vi "PosStrikerAnguloGol.vi"(8 "AnguloAttacker":dbl, 9 "atacando contra":bool, 10 "IA State":T1={"our_robots"=[], "enemy_robots"=[], "balls"=[], "geometry"={"line_width"=0, "field_length"=0, "field_width"=0, "boundary_width"=0, "referee_width"=0, "goal_width"=0, "goal_depth"=0, "goal_wall_width"=0, "center_circle_radius"=0, "defense_radius"=0, "defense_stretch"=0, "free_kick_from_defense_dist"=0, "penalty_spot_from_field_line_dist"=0, "penalty_line_from_spot_dist"=0}, "IA Judge"={"stage"="", "command"="", "our_goalie_id"=0.0, "enemy_goalie_id"=0.0, "command enum"=enum."Halt", "Time"=enum."Azul"}, "Received Timestamp"=timestamp(0 s since 1904-01-01), "Events"={"Touch"=FALSE, "Ball out"=FALSE, "id touch"=0.0, "Ball out of \nVision"=FALSE, "Ball inside \nGoalie area"=FALSE, "Robot not responding"=FALSE, "Robots responding status"=[1.0, 1.0, 1.0, 1.0, 1.0, 1.0], "Enemy Ball \nPossession"=FALSE, "Pass State"=FALSE, "id end of pass"=0.0, "Kick"=FALSE, "Id ini Possession"=0.0, "Ball Possesion"=FALSE, "Id Possesion"=0.0, "Direct Kick"=FALSE}}) -> (2 "theta final":dbl)   [LabVIEW 2017]
uses:
  Core/AI Input.ctl
  Core/AI Robot.ctl
  Intel/Functions Enum.ctl
  Intel/AttackerStates.ctl
  Path Planning/RRT/PathDests.ctl
  Path Planning/RRT/PathDest.ctl
  Core/AI Ball.ctl
  Core/Field Size.ctl
  Core/AI Judge.ctl
  Intel/Command Enum.ctl
  Events/Events.ctl
panel:
  in  "XdoAttacker":dbl
  in  "YdoAttacker":dbl
  in  "Array":dbl[](array[numeric])=[0.0, 0.0, 0.0, 0.0, 0.0, 0.0]
  in  "Contador 2":dbl
  in  "theta2":dbl=-1.57
  in  "inicio do intervalo":dbl=-1.57
  in  "tamanho do intervalo":dbl
  in  "valor de theta":dbl
  in  "RobôsParaAnalisar":dbl[][](array[numeric])=[[99999.0, 99999.0], [99999.0, 99999.0], [99999.0, 99999.0], [99999.0, 99999.0], [99999.0, 99999.0], [99999.0, 99999.0], [99999.0, 99999.0]]
  in  "Contador":dbl
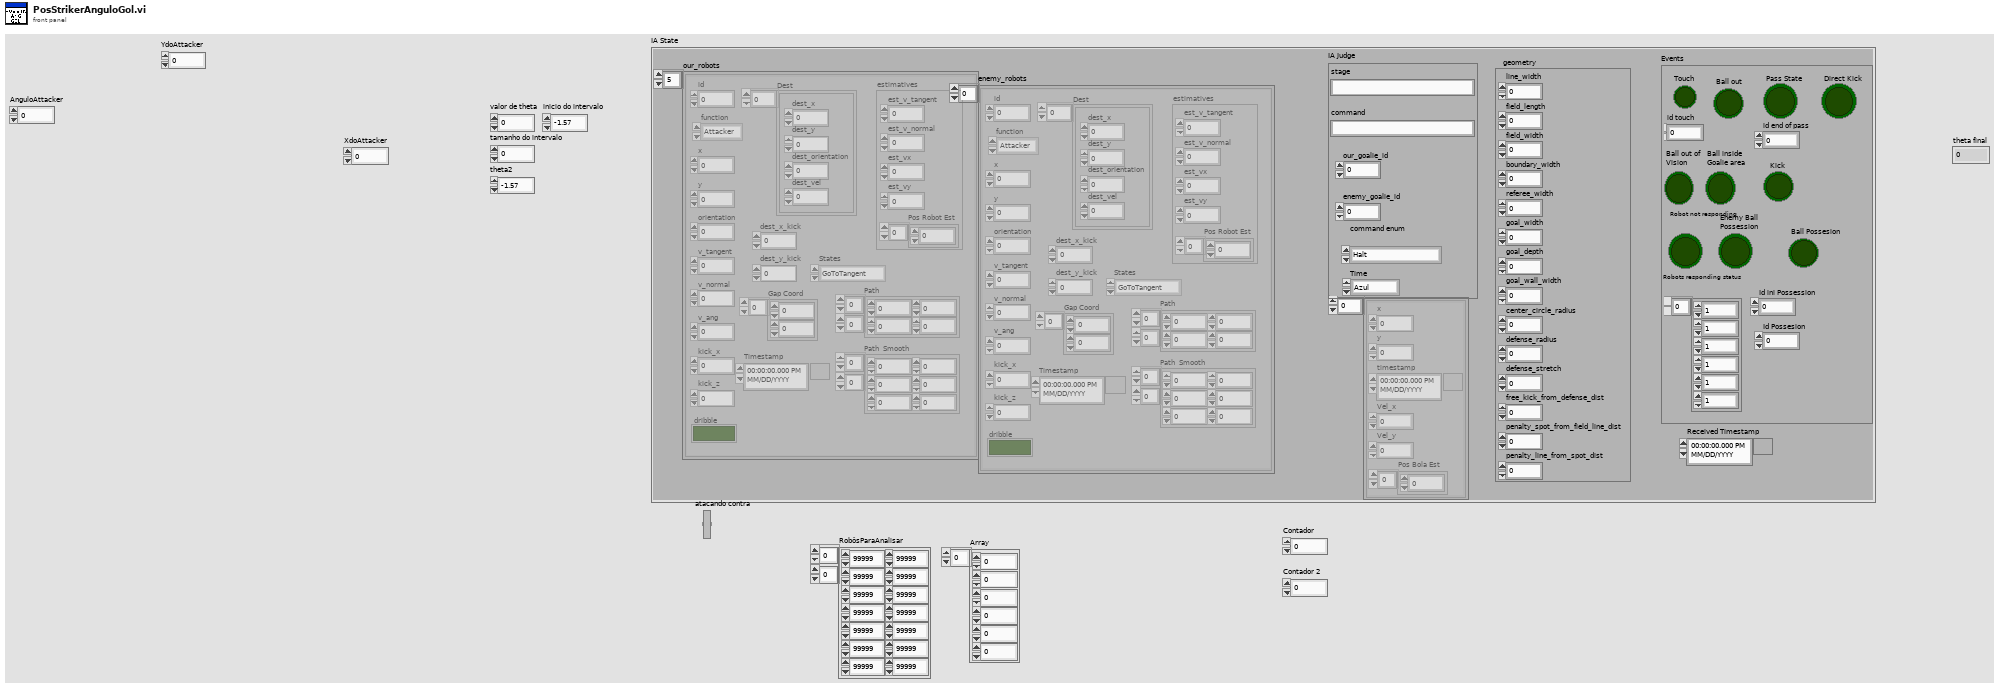
[diagram p1: front panel]
types:
  T1 = typedef "AI Input.ctl" = cluster{"our_robots":T2[], "enemy_robots":T2[], "balls":T7[], "geometry":T8, "IA Judge":T9, "Received Timestamp":timestamp, "Events":T11}
  T2 = typedef "AI Robot.ctl" = cluster{"id":u32, "function":T3, "x":dbl, "y":dbl, "orientation":dbl, "v_tangent":dbl, "v_normal":dbl, "v_ang":dbl, "kick_x":dbl, "kick_z":dbl, "dribble":bool, "Timestamp":timestamp, "estimatives":cluster{"est_v_tangent":dbl, "est_v_normal":dbl, "est_vx":dbl, "est_vy":dbl, "Pos Robot Est":dbl[]}, "dest_x_kick":dbl, "dest_y_kick":dbl, "Gap Coord":dbl[], "States":T4, "Path ":dbl[][], "Path  Smooth":dbl[][], "Dest":T5}
  T3 = typedef "Functions Enum.ctl" = enum16{"Attacker", "Goalie", "Defender", "Striker", "Goto 0", "Dummy", "Kicker", "ZigZag 0", "ZigZag 1", "ZigZag 2", "ZigZag 3", "ZigZag 4", "ZigZag 5", "ZigZag 6", "ZigZag 7", "ZigZag 8", ""}
  T4 = typedef "AttackerStates.ctl" = enum16{"Pass", "GoToTangent", "BallGetting", "GoToKick", ""}
  T5 = typedef "PathDests.ctl" = T6[]
  T6 = typedef "PathDest.ctl" = cluster{"dest_x":dbl, "dest_y":dbl, "dest_orientation":dbl, "dest_vel":dbl}
  T7 = typedef "AI Ball.ctl" = cluster{"x":dbl, "y":dbl, "timestamp":timestamp, "Vel_x":dbl, "Vel_y":dbl, "Pos Bola Est":dbl[]}
  T8 = typedef "Field Size.ctl" = cluster{"line_width":u32, "field_length":u32, "field_width":u32, "boundary_width":u32, "referee_width":u32, "goal_width":u32, "goal_depth":u32, "goal_wall_width":u32, "center_circle_radius":u32, "defense_radius":u32, "defense_stretch":u32, "free_kick_from_defense_dist":u32, "penalty_spot_from_field_line_dist":u32, "penalty_line_from_spot_dist":u32}
  T9 = typedef "AI Judge.ctl" = cluster{"stage":string, "command":string, "our_goalie_id":dbl, "enemy_goalie_id":dbl, "command enum":T10, "Time":enum16{"Azul", "Amarelo"}}
  T10 = typedef "Command Enum.ctl" = enum16{"Halt", "Stop", "Force Start", "PKA Normal Start", "Prepare Kickoff Ally", "PKE Normal Start", "Prepare Kickoff Enemy", "Prepare Penalty Ally", "PPA Normal Start", "Prepare Penalty Enemy", "PPE Normal Start", "Direct Free Enemy", "Direct Free Ally", "Indirect Free Enemy", "Indirect Free Ally", "Timeout Enemy", "Timeout Ally", "Goal Enemy", "Goal Ally", "Ball Placement Enemy", "Ball Placement Ally", "Normal Half Time", "Extra Time Break", "Extra Half Time", "None", "Post Game"}
  T11 = typedef "Events.ctl" = cluster{"Touch":bool, "Ball out":bool, "id touch":dbl, "Ball out of \nVision":bool, "Ball inside \nGoalie area":bool, "Robot not responding":bool, "Robots responding status":dbl[], "Enemy Ball \nPossession":bool, "Pass State":bool, "id end of pass":dbl, "Kick":bool, "Id ini Possession":dbl, "Ball Possesion":bool, "Id Possesion":dbl, "Direct Kick":bool}
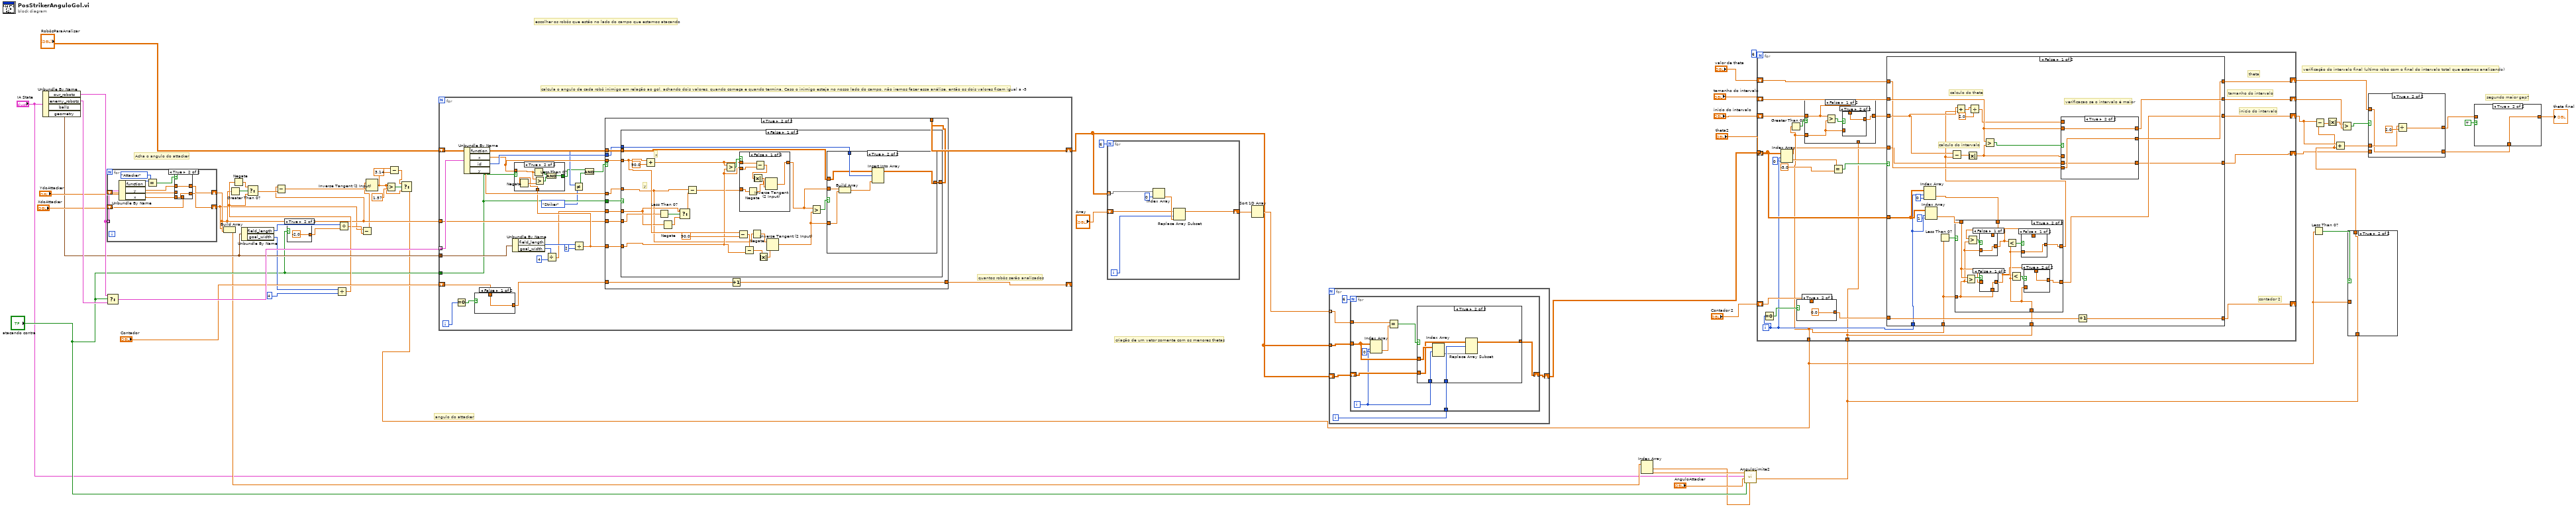
[diagram p0: block diagram]
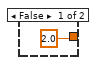
[diagram p4: hidden frame]
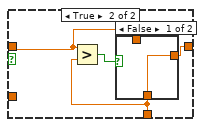
[diagram p9: hidden frame]
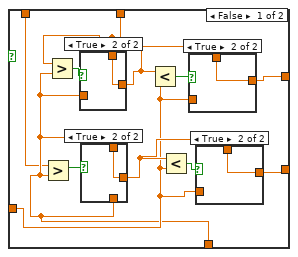
[diagram p12: hidden frame]
diagram:
  # "segundo maior gap?"
  # "verificação do intervalo final (ultimo robo com o final do intervalo total que estamos analisando)"
  # "calcula o angulo de cada robô inimigo em relação ao gol, achando dois valores, quando começa e quando termina. Caso o inimigo esteja no nosso lado do campo, não iremos fazer essa análise, então os dois valores ficam igual a -5"
  # "angulo do attacker"
  # "Acha o angulo do attacker"
  # "criação de um vetor somente com os menores thetas"
  # "escolher os robôs que estão no lado do campo que estamos atacando"
  n1 = Unbundle By Name("IA State") -> ("our_robots"=w37:T2[], "enemy_robots"=w60:T2[], "geometry"=w34:T8)  [unwired: 1 out]
  n2 = for {
    tunnel: w37 -> [w70] mode=indexing
    shift-right: [w65] -> w15
    shift-left: "YdoAttacker" -> [w64]
    shift-right: [w62] -> w14
    shift-left: "XdoAttacker" -> [w61]
    n3 = Unbundle By Name(w70) -> ("function"=w69:T3, "y"=w66:dbl, "x"=w63:dbl)
    n4 = Equal?(x=w69, y=Functions_Enum."Attacker") -> (x = y?=w67:bool)
    n5 = case shown="True" w67 {
      tunnel: w66 -> [_ w74]
      tunnel: [w72 w74] -> w65
      tunnel: w64 -> [w72 _]
      tunnel: w63 -> [_ w73]
      tunnel: [w71 w73] -> w62
      tunnel: w61 -> [w71 _]
      frame False {
      }
      frame True {
      }
    }
  }
  n6 = Select(t=w37, s="atacando contra", f=w60) -> (s? t:f=w59:T2[])
  n7 = Build Array(w14, w15) -> (w13:dbl[])
  n8 = Greater Than 0?(x=w15) -> (x > 0?=w30:bool)
  n9 = Unbundle By Name(w34) -> ("field_length"=w31:u32, "goal_width"=w33:u32)
  n10 = case shown="True" "atacando contra" {
    tunnel: [2.0 ("y") -2.0 ("y")] -> w25
    frame False {
    }
    frame True {
    }
  }
  n11 = Divide(x=w33, y=u32 4) -> (x/y=w28:dbl)
  n12 = Negate(x=w28) -> (-x=w29:dbl)
  n13 = Select(t=w29, s=w30, f=w28) -> (s? t:f=w27:dbl)
  n14 = Subtract(x=w15, y=w27) -> (x-y=w2:dbl)
  n15 = Divide(x=w31, y=w25) -> (x/y=w26:dbl)
  n16 = Subtract(x=w14, y=w26) -> (x-y=w1:dbl)
  n17 = Inverse Tangent (2 Input)(1:w2, 2:w1) -> (0:w4:dbl)
  n18 = Greater?(x=w4, y=1.57) -> (0:w7:bool)
  n19 = Subtract(x=w4, y=3.14) -> (x-y=w5:dbl)
  n20 = Select(t=w5, s=w7, f=w4) -> (s? t:f=w3:dbl)
  n21 = for {
    tunnel: w59 -> [w101] mode=indexing
    tunnel: "atacando contra" -> [w83]
    shift-right: [w91] -> w47
    shift-left: "RobôsParaAnalisar" -> [w100]
    shift-right: [w92] -> _
    shift-left: "Contador" -> [w94]
    tunnel: w34 -> [w84]
    tunnel: w15 -> [w88]
    i -> [w95]
    # "quantos robôs serão analisados"
    n22 = Equal To 0?(x=w95) -> (x = 0?=w96:bool)
    n23 = Unbundle By Name(w101) -> ("function"=w81:T3, "x"=w98:dbl, "id"=w99:u32, "y"=w97:dbl)
    n24 = case shown="False" w96 {
      tunnel: w94 -> [w102 _]
      tunnel: [w102 0.0] -> w93
      frame False {
      }
      frame True {
      }
    }
    n25 = Unbundle By Name(w84) -> ("field_length"=w90:u32, "goal_width"=w87:u32)
    n26 = Divide(x=w87, y=u32 4) -> (x/y=w85:dbl)
    n27 = Not Equal?(x=w81, y=Functions_Enum."Striker") -> (x != y?=w78:bool)
    n28 = Divide(x=w90, y=u32 2) -> (x/y=w89:dbl)
    n29 = case shown="True" w83 {
      tunnel: w98 -> [w108 w109]
      tunnel: [w104 w114] -> w77
      tunnel: w89 -> [w107 w110]
      frame False {
        n30 = Less?(x=w108, y=w107) -> (x < y?=w105:bool)
        n31 = Greater Than 0?(x=w108) -> (x > 0?=w106:bool)
        n32 = And(x=w106, y=w105) -> (x .and. y?=w104:bool)
      }
      frame True {
        n33 = Negate(x=w110) -> (-x=w111:dbl)
        n34 = Less Than 0?(x=w109) -> (x < 0?=w113:bool)
        n35 = Greater?(x=w109, y=w111) -> (0:w112:bool)
        n36 = And(x=w113, y=w112) -> (x .and. y?=w114:bool)
      }
    }
    n37 = And(x=w77, y=w78) -> (x .and. y?=w79:bool)
    n38 = case shown="True" w79 {
      tunnel: w100 -> [w119 w126]
      tunnel: w99 -> [w118 w124]
      tunnel: w98 -> [_ w128]
      tunnel: w97 -> [_ w125]
      tunnel: w93 -> [w120 w130]
      tunnel: [w120 w131] -> w92
      tunnel: [w115 w123] -> w91
      tunnel: w83 -> [_ w129]
      tunnel: w89 -> [_ w127]
      tunnel: w88 -> [_ w122]
      tunnel: w85 -> [_ w121]
      frame False {
        w117 = -5.0 ("element")
        n39 = Build Array(w117, w117) -> (w116:dbl[])
        n40 = Insert Into Array(array=w119, index (row)=w118, new element=w116) -> (w115:dbl[][])  [unwired: 1 in]
      }
      frame True {
        n41 = case shown="False" w129 {
          tunnel: w128 -> [w144 w193]
          tunnel: w127 -> [w143 w196]
          tunnel: w126 -> [w145 w188]
          tunnel: w125 -> [w133 w177]
          tunnel: w124 -> [w146 w187]
          tunnel: [w142 w184] -> w123
          tunnel: w122 -> [w137 w181]
          tunnel: w121 -> [w136 w178]
          frame False {
            # "y"
            # "x"
            n42 = Add(x=w144, y=90.0) -> (x+y=w152:dbl)
            n43 = Less Than 0?(x=w137) -> (x < 0?=w140:bool)
            n44 = Negate(x=w136) -> (-x=w139:dbl)
            n45 = Select(t=w136, s=w140, f=w139) -> (s? t:f=w138:dbl)
            n46 = Subtract(x=w133, y=w138) -> (x-y=w135:dbl)
            n47 = Greater?(x=w152, y=w143) -> (0:w153:bool)
            n48 = Subtract(x=w144, y=90.0) -> (x-y=w150:dbl)
            n49 = case shown="False" w153 {
              tunnel: w152 -> [w173 _]
              tunnel: [w171 1.57] -> w148
              tunnel: w143 -> [w172 _]
              tunnel: w135 -> [w167 _]
              frame False {
                n50 = Negate(x=w167) -> (-x=w168:dbl)
                n51 = Subtract(x=w173, y=w172) -> (x-y=w170:dbl)
                n52 = Absolute Value(x=w170) -> (abs(x)=w169:dbl)
                n53 = Inverse Tangent (2 Input)(1:w169, 2:w168) -> (0:w171:dbl)
              }
              frame True {
              }
            }
            n54 = Subtract(x=w150, y=w143) -> (x-y=w141:dbl)
            n55 = Negate(x=w133) -> (-x=w132:dbl)
            n56 = Absolute Value(x=w141) -> (abs(x)=w134:dbl)
            n57 = Inverse Tangent (2 Input)(1:w134, 2:w132) -> (0:w147:dbl)
            n58 = Greater?(x=w148, y=w147) -> (0:w149:bool)
            n59 = case shown="True" w149 {
              tunnel: w145 -> [w157 w163]
              tunnel: w146 -> [w159 w166]
              tunnel: w148 -> [w156 w164]
              tunnel: w147 -> [w158 w162]
              tunnel: [w155 w161] -> w142
              frame False {
                n60 = Build Array(w158, w156) -> (w160:dbl[])
                n61 = Insert Into Array(array=w157, index (row)=w159, new element=w160) -> (w155:dbl[][])  [unwired: 1 in]
              }
              frame True {
                n62 = Build Array(w164, w162) -> (w165:dbl[])
                n63 = Insert Into Array(array=w163, index (row)=w166, new element=w165) -> (w161:dbl[][])  [unwired: 1 in]
              }
            }
          }
          frame True {
            # "y"
            # "x"
            n64 = Negate(x=w196) -> (-x=w190:dbl)
            n65 = Subtract(x=w193, y=90.0) -> (x-y=w194:dbl)
            n66 = Greater Than 0?(x=w181) -> (x > 0?=w180:bool)
            n67 = Negate(x=w178) -> (-x=w179:dbl)
            n68 = Select(t=w178, s=w180, f=w179) -> (s? t:f=w176:dbl)
            n69 = Subtract(x=w177, y=w176) -> (x-y=w175:dbl)
            n70 = Less?(x=w194, y=w190) -> (x < y?=w195:bool)
            n71 = Add(x=w193, y=90.0) -> (x+y=w191:dbl)
            n72 = case shown="False" w195 {
              tunnel: w194 -> [w215 _]
              tunnel: [w212 1.57] -> w186
              tunnel: w190 -> [w214 _]
              tunnel: w175 -> [w213 _]
              frame False {
                n73 = Subtract(x=w215, y=w214) -> (x-y=w210:dbl)
                n74 = Absolute Value(x=w210) -> (abs(x)=w211:dbl)
                n75 = Inverse Tangent (2 Input)(1:w211, 2:w213) -> (0:w212:dbl)
              }
              frame True {
              }
            }
            n76 = Subtract(x=w191, y=w190) -> (x-y=w182:dbl)
            n77 = Absolute Value(x=w182) -> (abs(x)=w183:dbl)
            n78 = Inverse Tangent (2 Input)(1:w183, 2:w177) -> (0:w185:dbl)
            n79 = Greater?(x=w186, y=w185) -> (0:w189:bool)
            n80 = case shown="True" w189 {
              tunnel: w188 -> [w200 w206]
              tunnel: w187 -> [w202 w209]
              tunnel: w186 -> [w199 w207]
              tunnel: w185 -> [w201 w205]
              tunnel: [w198 w204] -> w184
              frame False {
                n81 = Build Array(w201, w199) -> (w203:dbl[])
                n82 = Insert Into Array(array=w200, index (row)=w202, new element=w203) -> (w198:dbl[][])  [unwired: 1 in]
              }
              frame True {
                n83 = Build Array(w207, w205) -> (w208:dbl[])
                n84 = Insert Into Array(array=w206, index (row)=w209, new element=w208) -> (w204:dbl[][])  [unwired: 1 in]
              }
            }
          }
        }
        n85 = Increment(x=w130) -> (x+1=w131:dbl)
      }
    }
  }
  n86 = for {
    N: 6 -> [_]
    tunnel: w47 -> [w222] mode=indexing
    shift-right: [w217] -> w49
    shift-left: "Array" -> [w218]
    i -> [w219]
    n87 = Index Array(array=w222, index=0) -> (element=w220:dbl)
    n88 = Replace Array Subset(array=w218, new element=w220, index=w219) -> (w217:dbl[])
  }
  n89 = Sort 1D Array(array=w49) -> (sorted array=w48:dbl[])
  n90 = for {
    tunnel: w48 -> [w225] mode=indexing
    tunnel: w47 -> [w227]
    shift-right: [w223] -> w46
    shift-left: w47 -> [w226]
    i -> [w224]
    n91 = for {
      N: 6 -> [_]
      tunnel: w227 -> [w233]
      shift-right: [w229] -> w223
      shift-left: w226 -> [w232]
      tunnel: w225 -> [w235]
      tunnel: w224 -> [w230]
      i -> [w231]
      n92 = Index Array(array=w233, index (row)=w231, index (col)=0 ("disabled index (col)")) -> (element=w236:dbl)
      n93 = Equal?(x=w235, y=w236) -> (x = y?=w234:bool)
      n94 = case shown="True" w234 {
        tunnel: w233 -> [_ w244]
        tunnel: w232 -> [w238 w240]
        tunnel: w231 -> [_ w243]
        tunnel: w230 -> [_ w242]
        tunnel: [w238 w239] -> w229
        frame False {
        }
        frame True {
          n95 = Index Array(array=w244, index (row)=w243) -> (element=w241:dbl[])  [unwired: 1 in]
          n96 = Replace Array Subset(array=w240, new element=w241, index (row)=w242) -> (w239:dbl[][])  [unwired: 1 in]
        }
      }
    }
  }
  n97 = Index Array(array=w13) -> (element #1=w11:dbl, element #2=w12:dbl)  [unwired: 2 in]
  n98 = call "AnguloLimite2.vi"("XdoAttacker"=w11, "atacando contra"="atacando contra", "AnguloAttacker"="AnguloAttacker", "IA State"="IA State", "YdoAttacker"=w12) -> ("Angulo Limite"=w9:dbl)  [unwired: 6 in]
  n99 = for {
    N: 6 -> [_]
    tunnel: w46 -> [w255]
    shift-right: [w263] -> w43
    shift-left: "valor de theta" -> [w264]
    shift-right: [w261] -> w45
    shift-left: "tamanho do intervalo" -> [w262]
    shift-right: [w260] -> w40
    shift-left: "inicio do intervalo" -> [w249]
    shift-right: [w256] -> _
    shift-left: "Contador 2" -> [w258]
    tunnel: w3 -> [w248]
    shift-right: [w246] -> w22
    shift-left: "theta2" -> [w247]
    tunnel: w9 -> [w245]
    i -> [w254]
    # "contador 2"
    # "inicio do intervalo"
    # "tamanho do intervalo"
    # "theta"
    n100 = Equal To 0?(x=w254) -> (x = 0?=w259:bool)
    n101 = Index Array(array=w255, index (row)=w254, index (col)=0 ("disabled index (col)")) -> (element=w253:dbl)
    n102 = Greater Than 0?(x=w248) -> (x > 0?=w251:bool)
    n103 = case shown="True" w259 {
      tunnel: w258 -> [w279 _]
      tunnel: [w279 0.0] -> w257
      frame False {
      }
      frame True {
      }
    }
    n104 = case shown="False" w251 {
      tunnel: [w269 w273] -> w250
      tunnel: w249 -> [w268 w275]
      tunnel: w248 -> [w267 _]
      tunnel: w245 -> [_ w274]
      frame False {
        n105 = Greater?(x=w268, y=w267) -> (0:w270:bool)
        n106 = case shown="True" w270 {
          tunnel: [w271 w272] -> w269
          tunnel: w268 -> [_ w272]
          tunnel: w267 -> [w271 _]
          frame False {
          }
          frame True {
          }
        }
      }
      frame True {
        n107 = Greater?(x=w275, y=w274) -> (0:w276:bool)
        n108 = case shown="False" w276 {
          tunnel: [w277 w278] -> w273
          tunnel: w275 -> [_ w278]
          tunnel: w274 -> [w277 _]
          frame False {
          }
          frame True {
          }
        }
      }
    }
    n109 = Equal?(x=w253, y=-5.0) -> (x = y?=w252:bool)
    n110 = case shown="False" w252 {
      tunnel: w264 -> [w290 w357]
      tunnel: [w291 w357] -> w263
      tunnel: w262 -> [w295 w356]
      tunnel: [w294 w356] -> w261
      tunnel: w250 -> [w306 w355]
      tunnel: [w284 w355] -> w260
      tunnel: w257 -> [w304 w354]
      tunnel: [w305 w354] -> w256
      tunnel: w255 -> [w303 _]
      tunnel: w254 -> [w302 _]
      tunnel: w248 -> [w288 _]
      tunnel: w247 -> [w283 w353]
      tunnel: [w282 w353] -> w246
      tunnel: w245 -> [w281 _]
      frame False {
        # "calculo do theta"
        # "calculo do intervalo"
        # "verificacao se o intervalo é maior"
        n111 = Index Array(array=w303, index (row)=w302, index (col)=0 ("disabled index (col)")) -> (element=w287:dbl)
        n112 = Index Array(array=w303, index (row)=w302, index (col)=1 ("disabled index (col)")) -> (element=w285:dbl)
        n113 = Less Than 0?(x=w288) -> (x < 0?=w289:bool)
        n114 = case shown="True" w289 {
          tunnel: w285 -> [w307 w335]
          tunnel: w287 -> [w308 w337]
          tunnel: w288 -> [w313 w334]
          tunnel: [w312 w332] -> w286
          tunnel: [w311 w328] -> w284
          tunnel: w281 -> [w310 w329]
          frame False {
            n115 = Greater?(x=w307, y=w310) -> (0:w317:bool)
            n116 = Greater?(x=w308, y=w310) -> (0:w318:bool)
            n117 = case shown="True" w318 {
              tunnel: [w325 w326] -> w309
              tunnel: w310 -> [w325 _]
              tunnel: w308 -> [_ w326]
              frame False {
              }
              frame True {
              }
            }
            n118 = case shown="True" w317 {
              tunnel: [w323 w324] -> w314
              tunnel: w310 -> [w323 _]
              tunnel: w310 -> [_ w324]
              frame False {
              }
              frame True {
              }
            }
            n119 = Less?(x=w309, y=w313) -> (x < y?=w316:bool)
            n120 = Less?(x=w314, y=w313) -> (x < y?=w315:bool)
            n121 = case shown="True" w316 {
              tunnel: [w321 w322] -> w312
              tunnel: w313 -> [w321 _]
              tunnel: w309 -> [_ w322]
              frame False {
              }
              frame True {
              }
            }
            n122 = case shown="True" w315 {
              tunnel: [w319 w320] -> w311
              tunnel: w314 -> [_ w320]
              tunnel: w313 -> [w319 _]
              frame False {
              }
              frame True {
              }
            }
          }
          frame True {
            n123 = Greater?(x=w335, y=w334) -> (0:w336:bool)
            n124 = Greater?(x=w337, y=w334) -> (0:w338:bool)
            n125 = case shown="False" w338 {
              tunnel: [w345 w346] -> w331
              tunnel: w337 -> [_ w346]
              tunnel: w334 -> [w345 _]
              frame False {
              }
              frame True {
              }
            }
            n126 = case shown="False" w336 {
              tunnel: w335 -> [_ w344]
              tunnel: [w343 w344] -> w327
              tunnel: w334 -> [w343 _]
              frame False {
              }
              frame True {
              }
            }
            n127 = Less?(x=w331, y=w329) -> (x < y?=w333:bool)
            n128 = Less?(x=w327, y=w329) -> (x < y?=w330:bool)
            n129 = case shown="False" w333 {
              tunnel: [w341 w342] -> w332
              tunnel: w331 -> [_ w342]
              tunnel: w329 -> [w341 _]
              frame False {
              }
              frame True {
              }
            }
            n130 = case shown="True" w330 {
              tunnel: [w339 w340] -> w328
              tunnel: w327 -> [_ w340]
              tunnel: w329 -> [w339 _]
              frame False {
              }
              frame True {
              }
            }
          }
        }
        n131 = Subtract(x=w306, y=w286) -> (x-y=w299:dbl)
        n132 = Add(x=w306, y=w286) -> (x+y=w298:dbl)
        n133 = Absolute Value(x=w299) -> (abs(x)=w293:dbl)
        n134 = Divide(x=w298, y=2.0) -> (x/y=w292:dbl)
        n135 = Greater?(x=w295, y=w293) -> (0:w296:bool)
        n136 = case shown="True" w296 {
          tunnel: w295 -> [_ w352]
          tunnel: [w349 w352] -> w294
          tunnel: w293 -> [w349 _]
          tunnel: w290 -> [w347 w351]
          tunnel: w292 -> [w348 _]
          tunnel: [w348 w351] -> w291
          tunnel: w283 -> [_ w350]
          tunnel: [w347 w350] -> w282
          frame False {
          }
          frame True {
          }
        }
        n137 = Increment(x=w304) -> (x+1=w305:dbl)
      }
      frame True {
      }
    }
  }
  n138 = Less Than 0?(x=w3) -> (x < 0?=w24:bool)
  n139 = case shown="True" w24 {
    tunnel: [w358 w359] -> w39
    tunnel: w3 -> [w358 _]
    tunnel: w9 -> [_ w359]
    frame False {
    }
    frame True {
    }
  }
  n140 = Subtract(x=w40, y=w39) -> (x-y=w42:dbl)
  n141 = Absolute Value(x=w42) -> (abs(x)=w41:dbl)
  n142 = Add(x=w40, y=w39) -> (x+y=w38:dbl)
  n143 = Greater?(x=w41, y=w45) -> (0:w44:bool)
  n144 = case shown="True" w44 {
    tunnel: [w361 w364] -> w18
    tunnel: w43 -> [w361 w362]
    tunnel: w38 -> [_ w363]
    tunnel: w22 -> [w360 _]
    tunnel: [w360 w362] -> w19
    frame False {
    }
    frame True {
      n145 = Divide(x=w363, y=2.0) -> (x/y=w364:dbl)
    }
  }
  n146 = case shown="True" TRUE {
    tunnel: [w366 w367] -> w20
    tunnel: w19 -> [_ w367]
    tunnel: w18 -> [w366 _]
    frame False {
    }
    frame True {
    }
  }
  "theta final" <- w20
